vi "Periodic Tasks.vi"(8 "error in":errorcluster) -> ()   [LabVIEW 2015]
doc: "This VI runs in parallel to other tasks. It can contain as many user-defined periodic loops as you need. These can carry out PID or other sorts of timed response."
uses:
  <vilib>/Rock Robotics/WPI/Utilities/WPI_GetSetVariantRefNum.vi
  <vilib>/Rock Robotics/Network Tables/NT Write Boolean.vi
  <vilib>/Rock Robotics/Network Tables/NT Write Number.vi
  Robot Global Data.vi
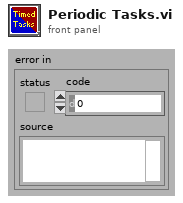
[diagram p1: front panel]
types:
  T1 = typedef "WPI_JoystickDevRef.ctl" = cluster{"Device":T2}
  T2 = typedef "WPI_JoystickDeviceEnum.ctl" = enum16{"USB 0", "USB 1", "USB 2", "USB 3", "USB 4", "USB 5"}
  T3 = typedef "WPI_RobotDriveDevRef.ctl" = cluster{"DevStatus":errorcluster, "Motors[]":T4[], "Square Inputs":bool, "Max Output":dbl}
  T4 = typedef "WPI_MotorControlDeviceRef.ctl" = cluster{"DeviceStatus":errorcluster, "Type":T5, "PWM":cluster{"PWM Channel":T6, "DeadBand":T7}, "CAN":cluster{"Device Number":u8, "Control Mode":T8, "Semaphore":T9, "Max Vout":dbl, "TalonSRX Control Mode":T10}, "Invert":bool}
  T5 = typedef "WPI_MotorControlType.ctl" = enum16{"PWM", "CAN", "CANTalonSRX"}
  T6 = typedef "FPGA_DIOPWMChannel.ctl" = enum8{"PWM 0", "PWM 1", "PWM 2", "PWM 3", "PWM 4", "PWM 5", "PWM 6", "PWM 7", "PWM 8", "PWM 9", "PWM MXP 0", "PWM MXP 1", "PWM MXP 2", "PWM MXP 3", "PWM MXP 4", "PWM MXP 5", "PWM MXP 6", "PWM MXP 7", "PWM MXP 8", "PWM MXP 9", "Invalid"}
  T7 = typedef "WPI_PWMDeadband.ctl" = cluster{"Name":string, "maxPositivePwm":i32, "minPositivePwm":i32, "centerPwm":i32, "maxNegativePwm":i32, "minNegativePwm":i32, "angularRange":u16}
  T8 = typedef "WPI_CANJaguar_ControlMode.ctl" = enum8{"Percent VBus", "Current", "Speed", "Position", "Voltage"}
  T9 = typedef "Semaphore RefNum" = refnum<k1>
  T10 = typedef "WPI_CANTalonSRX_APIControlMode.ctl" = enum8{"Percent VBus", "Speed", "Position", "Slave", "Unchanged / Invalid", "Voltage Compensation", "Current", "Motion Profile"}
  T11 = typedef "WPI_DigitalInputDevRef.ctl" = cluster{"DevStatus":errorcluster, "DIO Channel":T12}
  T12 = typedef "FPGA_DIOChannel.ctl" = enum8{"DIO 0", "DIO 1", "DIO 2", "DIO 3", "DIO 4", "DIO 5", "DIO 6", "DIO 7", "DIO 8", "DIO 9", "DIO MXP 0", "DIO MXP 1", "DIO MXP 2", "DIO MXP 3", "DIO MXP 4", "DIO MXP 5", "DIO MXP 6", "DIO MXP 7", "DIO MXP 8", "DIO MXP 9", "DIO MXP 10", "DIO MXP 11", "DIO MXP 12", "DIO MXP 13", "DIO MXP 14", "DIO MXP 15", "Invalid"}
  T13 = typedef "WPI_EncoderDevRef.ctl" = cluster{"DevStatus":errorcluster, "EncoderIndex":T14, "CounterIndex":T15, "DistancePerCount":dbl, "Decoding Type":T16}
  T14 = typedef "FPGA_EncoderIdx.ctl" = enum8{"Enc 0", "Enc 1", "Enc 2", "Enc 3", "Enc 4", "Enc 5", "Enc 6", "Enc 7", "Invalid"}
  T15 = typedef "FPGA_CounterCtrSystemIndex.ctl" = enum8{"Ctr 0", "Ctr 1", "Ctr 2", "Ctr 3", "Ctr 4", "Ctr 5", "Ctr 6", "Ctr 7", "Invalid"}
  T16 = typedef "WPI_EncoderType.ctl" = enum16{"1x", "2x", "4x"}
  T17 = typedef "WPI_GyroDevRef.ctl" = cluster{"DevStatus":errorcluster, "Analog Channel":T18, "Offset":dbl, "Gain (VoltsPerDegree/Second)":dbl, "Gyro Type":enum16{"Analog", "XRS450"}, "Handle":i32, "SPI Bus":T19, "Device Found":bool, "Sample Rate":dbl, "Calibrate On Open":bool}
  T18 = typedef "FPGA_AIChannel.ctl" = enum8{"AI 0", "AI 1", "AI 2", "AI 3", "AI MXP 0", "AI MXP 1", "AI MXP 2", "AI MXP 3", "Invalid"}
  T19 = typedef "spi_bus.ctl" = enum16{"SPI On-Board, CS0", "SPI On-Board, CS1", "SPI On-Board, CS2", "SPI On-Board, CS3", "SPI MXP", "Invalid"}
  T20 = cluster{"JoystickDevRef":T1, "RobotDriveDevRef":T3}
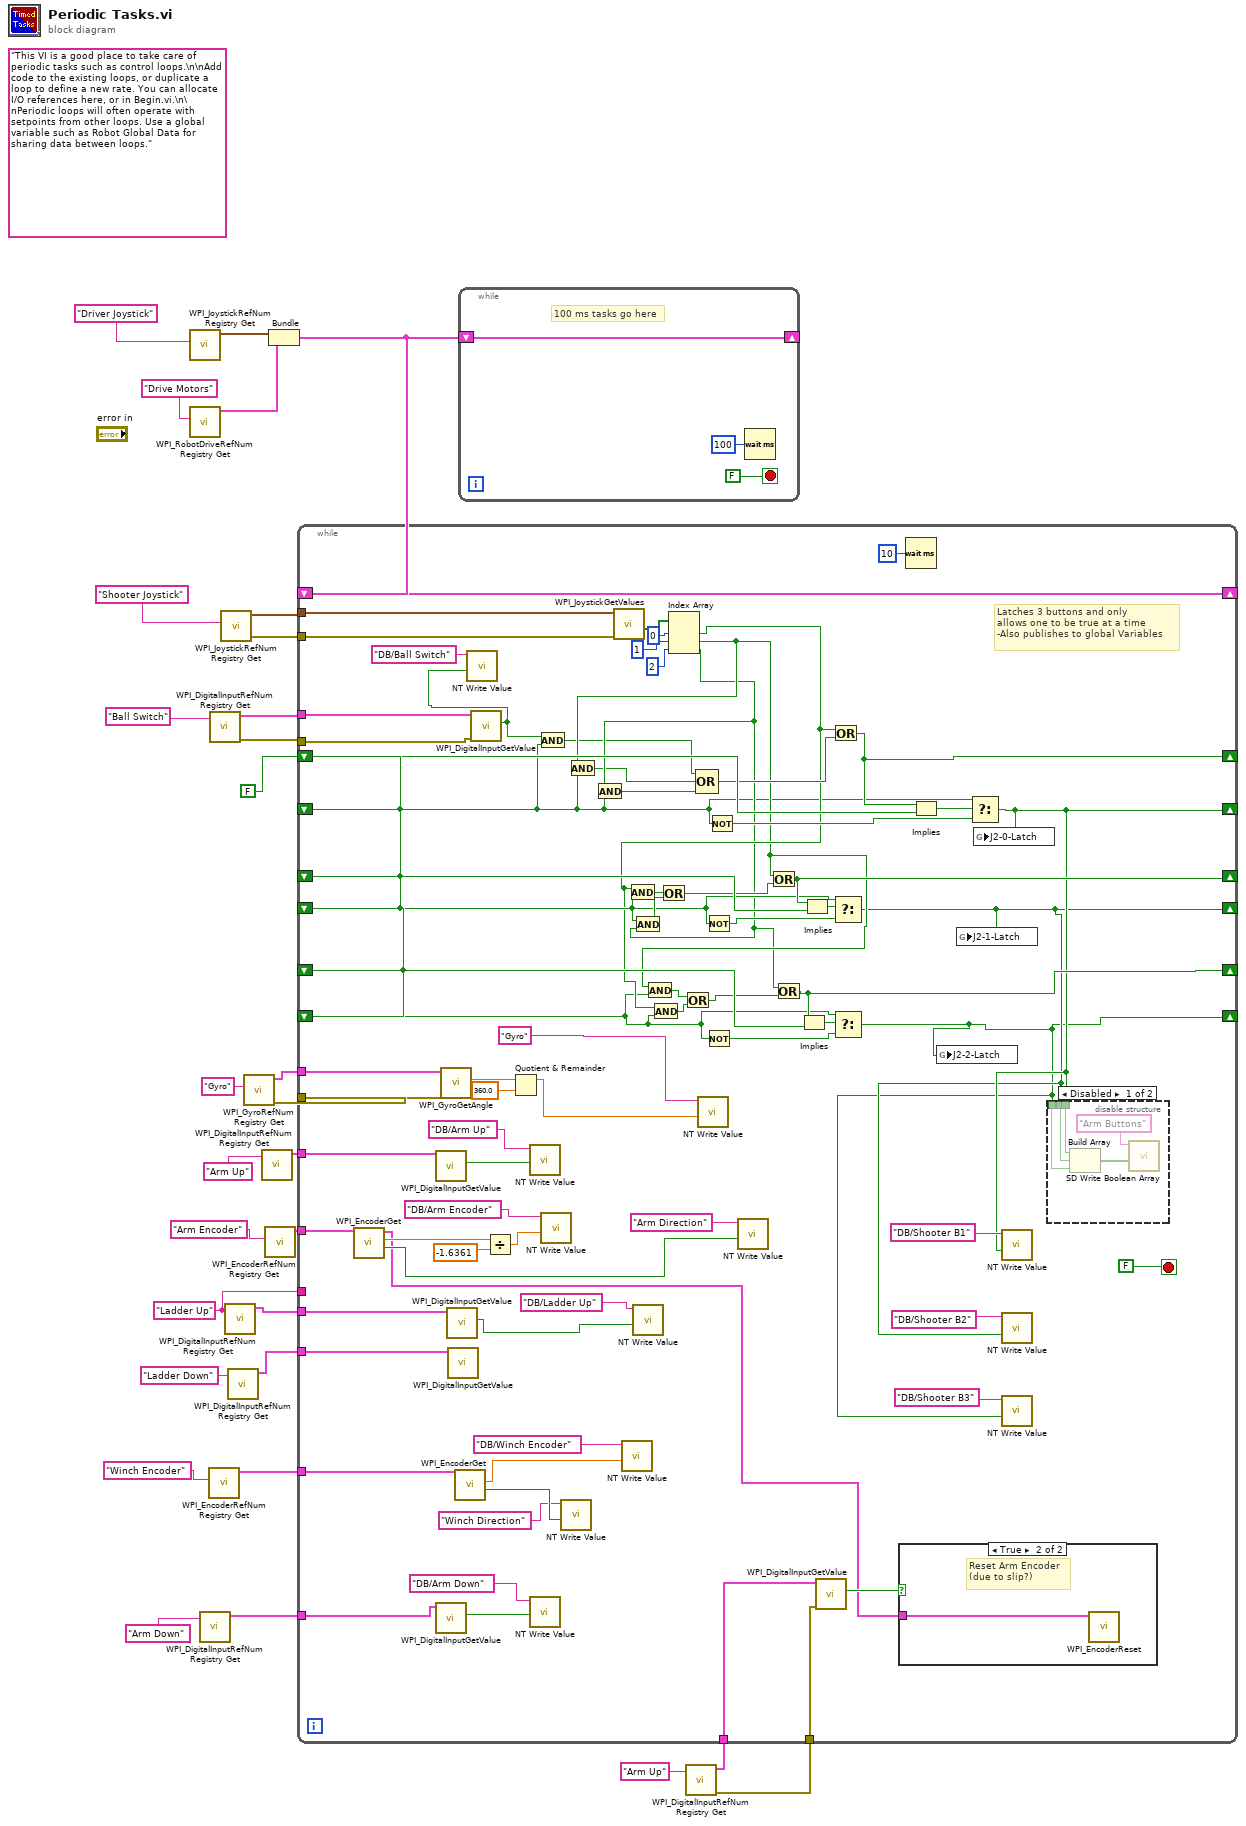
[diagram p0: block diagram]
diagram:
  w12 = "Ladder Up" ("refnum name")
  w21 = FALSE ("button 1")
  (unwired) "This VI is a good place to take care of periodic tasks such as control loops.\n\nAdd code to the existing loops, or duplicate a loop to define a new rate. You can allocate I/O references here, or in Begin.vi.\n\nPeriodic loops will often operate with setpoints from other loops. Use a global variable such as Robot Global Data for sharing data between loops."
  n1 = call <vilib>:"WPI_JoystickRefNum Registry Get.vi"("refnum name"="Driver Joystick") -> ("JoystickDevRef"=w28:T1)  [unwired: 1 in, 9 out]
  n2 = call <vilib>:"WPI_RobotDriveRefNum Registry Get.vi"("refnum name"="Drive Motors") -> ("RobotDriveDevRef"=w27:T3)  [unwired: 1 in, 9 out]
  n3 = call <vilib>:"WPI_DigitalInputRefNum Registry Get.vi"("refnum name"="Arm Down") -> ("DigitalInputDevRef"=w4:T11)  [unwired: 9 in, 1 out]
  n4 = call <vilib>:"WPI_EncoderRefNum Registry Get.vi"("refnum name"="Winch Encoder") -> ("EncoderDevRef"=w8:T13)  [unwired: 9 in, 1 out]
  n5 = call <vilib>:"WPI_DigitalInputRefNum Registry Get.vi"("refnum name"="Ball Switch") -> ("error out"=w22:errorcluster, "DigitalInputDevRef"=w23:T11)  [unwired: 9 in]
  n6 = call <vilib>:"WPI_JoystickRefNum Registry Get.vi"("refnum name"="Shooter Joystick") -> ("error out"=w18:errorcluster, "JoystickDevRef"=w19:T1)  [unwired: 1 in, 8 out]
  n7 = call <vilib>:"WPI_DigitalInputRefNum Registry Get.vi"("refnum name"=w12) -> ("DigitalInputDevRef"=w14:T11)  [unwired: 9 in, 1 out]
  n8 = call <vilib>:"WPI_DigitalInputRefNum Registry Get.vi"("refnum name"="Ladder Down") -> ("DigitalInputDevRef"=w13:T11)  [unwired: 9 in, 1 out]
  n9 = call <vilib>:"WPI_GyroRefNum Registry Get.vi"("refnum name"="Gyro") -> ("error out"=w24:errorcluster, "GyroDevRef"=w25:T17)  [unwired: 9 in]
  n10 = call <vilib>:"WPI_DigitalInputRefNum Registry Get.vi"("refnum name"="Arm Up") -> ("DigitalInputDevRef"=w7:T11)  [unwired: 9 in, 1 out]
  n11 = call <vilib>:"WPI_EncoderRefNum Registry Get.vi"("refnum name"="Arm Encoder") -> ("EncoderDevRef"=w16:T13)  [unwired: 9 in, 1 out]
  n12 = Bundle("JoystickDevRef"=w28, "RobotDriveDevRef"=w27) -> (w17:T20)  [unwired: 1 out]
  n13 = while {
    shift-right: [w31] -> _
    shift-left: w17 -> [w31]
    stop <- FALSE stop-if-true
    # "100 ms tasks go here"
    n14 = Wait (ms)(milliseconds to wait=u32 100) -> ()  [unwired: 1 out]
  }
  n15 = call <vilib>:"WPI_DigitalInputRefNum Registry Get.vi"("refnum name"="Arm Up") -> ("error out"=w1:errorcluster, "DigitalInputDevRef"=w2:T11)  [unwired: 9 in]
  n16 = while {
    shift-right: [w92] -> _
    shift-left: w21 -> [w110]
    shift-right: [w44] -> _
    shift-left: w21 -> [w74]
    shift-right: [w101] -> _
    shift-left: w21 -> [w105]
    shift-right: [w43] -> _
    shift-left: w21 -> [w97]
    shift-right: [w96] -> _
    shift-left: w21 -> [w102]
    shift-right: [w90] -> _
    shift-left: w17 -> [w90]
    tunnel: w19 -> [w82]
    tunnel: w25 -> [w79]
    tunnel: w24 -> [w78]
    shift-right: [w42] -> _
    shift-left: w21 -> [w77]
    tunnel: w23 -> [w76]
    tunnel: w22 -> [w75]
    tunnel: w18 -> [w70]
    tunnel: w16 -> [w67]
    tunnel: w14 -> [w66]
    tunnel: w13 -> [w65]
    tunnel: w12 -> [_]
    tunnel: w8 -> [w63]
    tunnel: w7 -> [w58]
    tunnel: w4 -> [w56]
    tunnel: w2 -> [w37]
    tunnel: w1 -> [w36]
    stop <- FALSE ("stop") stop-if-true
    # "Latches 3 buttons and only\nallows one to be true at a time\n-Also publishes to global Variables"
    n17 = call <vilib>:"WPI_EncoderGet.vi"("EncoderDevRef"=w67) -> ("Direction"=w40:bool, "Distance"=w54:dbl, "EncoderDevRef"=w34:T13)  [unwired: 5 in, 3 out]
    n18 = call <vilib>:"WPI_DigitalInputGetValue.vi"("DigitalInputDevRef"=w58) -> ("Value"=w52:bool)  [unwired: 8 in, 2 out]
    n19 = call <vilib>:"WPI_DigitalInputGetValue.vi"("DigitalInputDevRef"=w56) -> ("Value"=w57:bool)  [unwired: 8 in, 2 out]
    n20 = call <vilib>:"WPI_GyroGetAngle.vi"("error in"=w78, "GyroDevRef"=w79) -> ("Angle"=w81:dbl)  [unwired: 5 in, 4 out]
    n21 = call <vilib>:"WPI_DigitalInputGetValue.vi"("DigitalInputDevRef"=w66) -> ("Value"=w64:bool)  [unwired: 8 in, 2 out]
    n22 = call <vilib>:"WPI_DigitalInputGetValue.vi"("DigitalInputDevRef"=w65) -> ()  [unwired: 8 in, 3 out]
    n23 = call <vilib>:"WPI_EncoderGet.vi"("EncoderDevRef"=w63) -> ("Direction"=w62:bool, "Distance"=w60:dbl)  [unwired: 5 in, 4 out]
    n24 = call <vilib>:"WPI_DigitalInputGetValue.vi"("error in (no error)"=w75, "DigitalInputDevRef"=w76) -> ("Value"=w39:bool)  [unwired: 7 in, 2 out]
    n25 = call-poly <vilib>:"NT Write Value.vi"("Boolean"=w39, "Name"="DB/Ball Switch") -> ()  [unwired: 9 in, 1 out]
    n26 = Divide(x=w54, y=-1.6361 ("Arm Calibration")) -> (x/y=w53:dbl)
    n27 = Quotient & Remainder(x=w81, y=360.0) -> (x-y*floor(x/y)=w68:dbl)  [unwired: 1 out]
    n28 = call-poly <vilib>:"NT Write Value.vi"("Boolean"=w52, "Name"="DB/Arm Up") -> ()  [unwired: 9 in, 1 out]
    n29 = call-poly <vilib>:"NT Write Value.vi"("Boolean"=w57, "Name"="DB/Arm Down") -> ()  [unwired: 9 in, 1 out]
    n30 = And(x=w39, y=w74) -> (x .and. y?=w73:bool)
    n31 = call-poly <vilib>:"NT Write Value.vi"("Numeric"=w53, "Name"="DB/Arm Encoder") -> ()  [unwired: 9 in, 1 out]
    n32 = call-poly <vilib>:"NT Write Value.vi"("Boolean"=w62, "Name"="Winch Direction") -> ()  [unwired: 9 in, 1 out]
    n33 = call <vilib>:"WPI_JoystickGetValues.vi"("error in (no error)"=w70, "JoystickDevRef"=w82) -> ("Buttons"=w89:bool[])  [unwired: 5 in, 4 out]
    n34 = call-poly <vilib>:"NT Write Value.vi"("Numeric"=w60, "Name"="DB/Winch Encoder") -> ()  [unwired: 9 in, 1 out]
    n35 = call-poly <vilib>:"NT Write Value.vi"("Boolean"=w64, "Name"="DB/Ladder Up") -> ()  [unwired: 9 in, 1 out]
    n36 = Index Array(array=w89, index #1=0 ("index"), index #2=1 ("index"), index #3=2 ("index")) -> (element #1=w85:bool, element #2=w84:bool, element #3=w83:bool)
    n37 = And(x=w84, y=w74) -> (x .and. y?=w72:bool)
    n38 = And(x=w83, y=w74) -> (x .and. y?=w71:bool)
    n39 = And(x=w85, y=w97) -> (x .and. y?=w99:bool)
    n40 = And(x=w97, y=w83) -> (x .and. y?=w98:bool)
    n41 = And(x=w84, y=w77) -> (x .and. y?=w94:bool)
    n42 = And(x=w85, y=w77) -> (x .and. y?=w93:bool)
    n43 = Or(x=w99, y=w98) -> (x .or. y?=w100:bool)
    n44 = Or(x=w94, y=w93) -> (x .or. y?=w95:bool)
    n45 = Compound Arithmetic op=OR(w73, w72, w71) -> (w91:bool)
    n46 = call-poly <vilib>:"NT Write Value.vi"("Numeric"=w68, "Name"="Gyro") -> ()  [unwired: 9 in, 1 out]
    n47 = Not(x=w97) -> (.not. x?=w107:bool)
    n48 = Not(x=w77) -> (.not. x?=w103:bool)
    n49 = Not(x=w74) -> (.not. x?=w112:bool)
    n50 = call-poly <vilib>:"NT Write Value.vi"("Boolean"=w40, "Name"="Arm Direction") -> ()  [unwired: 9 in, 1 out]
    n51 = Or(x=w84, y=w100) -> (x .or. y?=w101:bool)
    n52 = Or(x=w83, y=w95) -> (x .or. y?=w96:bool)
    n53 = Implies(1:w102, 2:w96) -> (0:w104:bool)
    n54 = Implies(1:w105, 2:w101) -> (0:w106:bool)
    n55 = call <vilib>:"WPI_DigitalInputGetValue.vi"("error in (no error)"=w36, "DigitalInputDevRef"=w37) -> ("Value"=w35:bool)  [unwired: 7 in, 2 out]
    n56 = Or(x=w85, y=w91) -> (x .or. y?=w92:bool)
    n57 = Select(t=w97, s=w106, f=w107) -> (s? t:f=w43:bool)
    n58 = Select(t=w77, s=w104, f=w103) -> (s? t:f=w42:bool)
    n59 = case shown="True" w35 {
      tunnel: w34 -> [_ w113]
      frame False {
      }
      frame True {
        # "Reset Arm Encoder\n(due to slip?)"
        n60 = call <vilib>:"WPI_EncoderReset.vi"("EncoderDevRef"=w113) -> ()  [unwired: 9 in, 2 out]
      }
    }
    n61 = Wait (ms)(milliseconds to wait=u32 10) -> ()  [unwired: 1 out]
    n62 = Implies(1:w110, 2:w92) -> (0:w111:bool)
    n63 = global write "Robot Global Data.vi" "J2-2-Latch"(w42) -> ()
    n64 = global write "Robot Global Data.vi" "J2-1-Latch"(w43) -> ()
    n65 = Select(t=w74, s=w111, f=w112) -> (s? t:f=w44:bool)
    n66 = global write "Robot Global Data.vi" "J2-0-Latch"(w44) -> ()
    n67 = call-poly <vilib>:"NT Write Value.vi"("Boolean"=w44, "Name"="DB/Shooter B1") -> ()  [unwired: 9 in, 1 out]
    n68 = call-poly <vilib>:"NT Write Value.vi"("Boolean"=w43, "Name"="DB/Shooter B2") -> ()  [unwired: 9 in, 1 out]
    n69 = call-poly <vilib>:"NT Write Value.vi"("Boolean"=w42, "Name"="DB/Shooter B3") -> ()  [unwired: 9 in, 1 out]
    n70 = disable-structure shown="Disabled" {
      disable-tunnel: w43 -> [w116 _]
      disable-tunnel: w44 -> [w115 _]
      disable-tunnel: w42 -> [w114 _]
      frame Disabled {
        n71 = Build Array(w115, w116, w114) -> (w118:bool[])
        n72 = call <vilib>:"SD Write Boolean Array.vi"("Boolean Array"=w118, "Name"="Arm Buttons") -> ()  [unwired: 8 in, 2 out]
      }
      frame Enabled {
      }
    }
  }
